vi "Sound File to Sound Output.vi"() -> ()   [LabVIEW 2023]
doc: "This VI illustrates how to play a sound file continuously, reading the sound file in pieces, and playing each piece at a time."
uses:
  <vilib>/sound2/lvsound2.llb/Sampling Mode.ctl
  <vilib>/Analysis/3filter.llb/Filter Passband Type.ctl
  <vilib>/sound2/lvsound2.llb/Sound File Info (path).vi
  <vilib>/sound2/lvsound2.llb/Sound File Read Open.vi
  <vilib>/sound2/lvsound2.llb/Sound File Read (DBL).vi
  <vilib>/sound2/lvsound2.llb/Sound Output Write (DBL).vi
  <vilib>/Analysis/3filter.llb/Butterworth Filter (DBL).vi
  <vilib>/Analysis/NI_AALBase.lvlib
panel:
  out "sample rate (S/s)":dbl
  in  "low cutoff freq: fl":dbl=0.12500000000000006 format="%0.4f"
  in  "path":path
  out "Current Data":waveform(dbl)[](graph)
  out "Current Iteration":i32
  in  "Stop":bool
  in  "Number of Samples/Iteration":i32=2500
  in  "Device ID":u32
  # "Overview: Demonstrates the use of the Sound VIs to play a sound file continuously, reading the sound file in pieces, and playing each piece one at a time.\nInstructions:\n1. Specify the Device ID and the Number of Samples/Iteration.\n2. Run the VI."
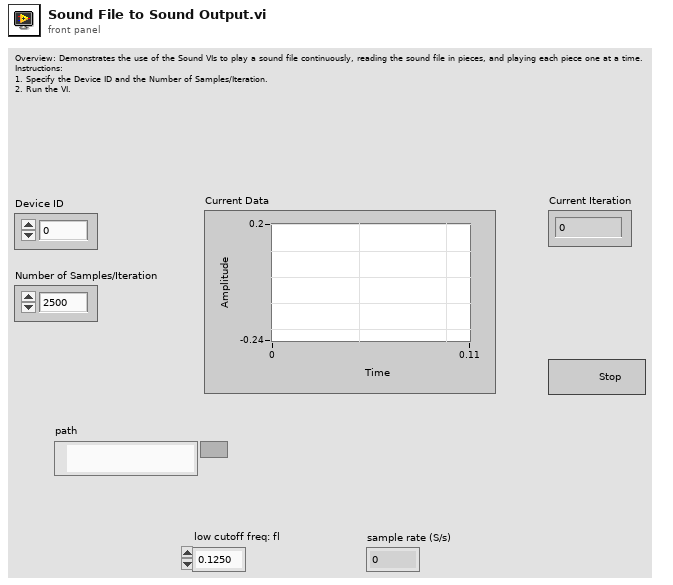
[diagram p1: front panel]
types:
  T1 = typedef "Sampling Mode.ctl" = i32
  T2 = typedef "Sound Data Format.ctl" = cluster{"sample rate (S/s)":dbl, "number of channels":i32, "bits per sample":i32}
  T3 = typedef "Sound File Refnum.ctl" = refnum<file>
  T4 = typedef "Sound Output Task ID.ctl" = u32
  T5 = typedef "NI_AALBase.lvlib/Filter Passband Type.ctl" = enum32{"Lowpass", "Highpass", "Bandpass", "Bandstop"}
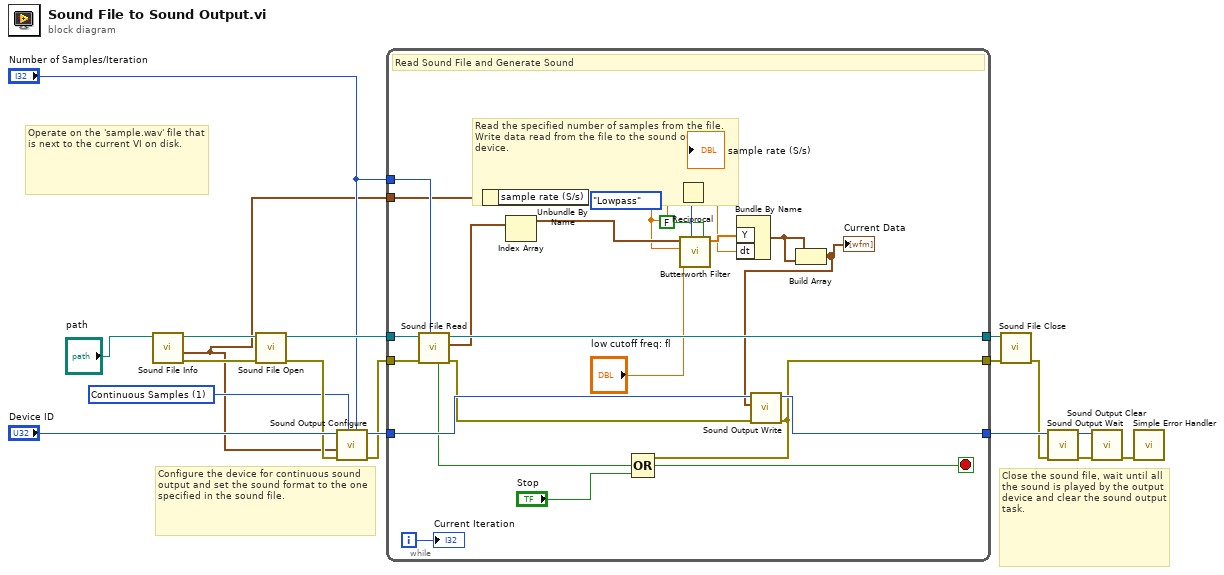
[diagram p0: block diagram]
diagram:
  w4 = T1 1 items=["Finite Samples", "Continuous Samples"] ("sample mode")
  # "Operate on the 'sample.wav' file that is next to the current VI on disk."
  # "Close the sound file, wait until all the sound is played by the output device and clear the sound output task."
  # "Configure the device for continuous sound output and set the sound format to the one specified in the sound file."
  n1 = call-poly <vilib>:"Sound File Info.vi"("path"="path") -> ("error out"=w13:errorcluster, "sound format"=w1:T2, "path out"=w6:path)  [unwired: 7 in, 1 out]
  n2 = call-poly <vilib>:"Sound File Open.vi"("error in (no error)"=w13, "path"=w6) -> ("error out"=w12:errorcluster, "sound file refnum"=w14:T3)  [unwired: 8 in]
  n3 = call <vilib>:"Sound Output Configure.vi"("number of samples/ch"="Number of Samples/Iteration", "sample mode"=w4, "error in (no error)"=w12, "sound format"=w1, "device ID"="Device ID") -> ("error out"=w11:errorcluster, "task ID"=w18:T4)  [unwired: 5 in]
  n4 = while {
    tunnel: "Number of Samples/Iteration" -> [w31]
    tunnel: w14 -> [w39]
    tunnel: [w37] -> w16
    tunnel: w11 -> [w40]
    tunnel: [w30] -> w15
    tunnel: w18 -> [w36]
    tunnel: [w41] -> w9
    tunnel: w1 -> [w27]
    i -> [w38]
    stop <- w32 stop-if-true
    # "Read the specified number of samples from the file. Write data read from the file to the sound output device."
    # "Read Sound File and Generate Sound"
    n5 = call-poly <vilib>:"Sound File Read.vi"("number of samples/ch (-1: all)"=w31, "error in (no error)"=w40, "sound file refnum"=w39) -> ("error out"=w35:errorcluster, "data"=w29:waveform(dbl)[], "sound file refnum out"=w37:T3, "end of file?"=w33:bool)  [unwired: 4 in, 1 out]
    n6 = Unbundle By Name(w27) -> ("sample rate (S/s)"=w23:dbl)
    "sample rate (S/s)" <- w23
    n7 = Index Array(array=w29) -> (element=w28:waveform(dbl))  [unwired: 1 in]
    n8 = Reciprocal(x=w23) -> (1/x=w22:dbl)
    n9 = call-poly <vilib>:"Butterworth Filter.vi"("init/cont (init:F)"=FALSE, "filter type"=Filter_Passband_Type."Lowpass", "low cutoff freq: fl"="low cutoff freq: fl", "sampling freq: fs"=w23, "X"=w28) -> ("Filtered X"=w24:dbl[])  [unwired: 3 in, 1 out]
    n10 = Bundle By Name("Y"=w24, "dt"=w22) -> (w21:waveform(dbl))  [unwired: 1 in]
    n11 = Build Array(w21, w21) -> (w20:waveform(dbl)[])
    "Current Data" <- w20
    n12 = call-poly <vilib>:"Sound Output Write.vi"("error in (no error)"=w35, "data"=w20, "task ID"=w36) -> ("error out"=w30:errorcluster, "task ID out"=w41:T4)  [unwired: 7 in]
    n13 = Compound Arithmetic op=OR(w30, w33, "Stop") -> (w32:bool)
    "Current Iteration" <- w38
  }
  n14 = call <vilib>:"Sound File Close.vi"("error in (no error)"=w15, "sound file refnum"=w16) -> ("error out"=w8:errorcluster)  [unwired: 9 in]
  n15 = call <vilib>:"Sound Output Wait.vi"("error in (no error)"=w8, "task ID"=w9) -> ("error out"=w7:errorcluster, "task ID out"=w10:T4)  [unwired: 8 in]
  n16 = call <vilib>:"Sound Output Clear.vi"("error in (no error)"=w7, "task ID"=w10) -> ("error out"=w3:errorcluster)  [unwired: 9 in]
  n17 = call <vilib>:"Simple Error Handler.vi"("error in (no error)"=w3) -> ()  [unwired: 4 in, 5 out]
